vi "Generate Model.vi"(8 "error in (no error)":errorcluster, 11 "Velodyne 3D LIDAR in":refnum<class "Velodyne 3D LIDAR.lvclass">) -> (0 "error out":errorcluster, 3 "Velodyne 3D LIDAR out":refnum<class "Velodyne 3D LIDAR.lvclass">)   [LabVIEW 2017, in "NI_Robotics_Simulator.lvlib" / "Velodyne 3D LIDAR.lvclass"]
uses:
  <vilib>/robotics/Simulator/Plugin/Sensor/Velodyne 3D LIDAR/Velodyne 3D LIDAR.lvclass
  <vilib>/robotics/Simulator/Plugin/Sensor/Velodyne 3D LIDAR/Velodyne 3D LIDAR.lvclass/Velodyne 3D LIDAR.ctl
  <vilib>/robotics/Simulator/Robot Factory/Sensor/Base/ODESimulator_Base_Sensor.lvclass
  <vilib>/robotics/Simulator/3D-Physics/Sphere/3D_Physics_Sphere.lvclass
  c:/Program Files (x86)/National Instruments/LabVIEW 2017/vi.lib/robotics/Simulator/3D-Physics/Base/3D_Physics_Base.lvclass
  <vilib>/Utility/miscctls.llb/LV3DPointTypeDef.ctl
  <vilib>/robotics/Simulator/Robot Factory/Motor/ctl/Rate Joint.ctl
  <vilib>/robotics/Simulator/Robot Factory/Joint/Utilities/Joint Axis.ctl
  <vilib>/robotics/Simulator/Robot Factory/Motor/ODESimulator_Motor.lvclass
  <vilib>/Utility/xml.llb/Read From XML File(string).vi
  <vilib>/robotics/Simulator/3D-Physics/Base/3D_Physics_Base.lvclass
  <vilib>/robotics/Simulator/Robot Factory/Sensor/LIDAR/ODESimulator_LIDAR.lvclass
  <vilib>/robotics/Simulator/Robot Factory/Joint/ODESimulator_Joint.lvclass
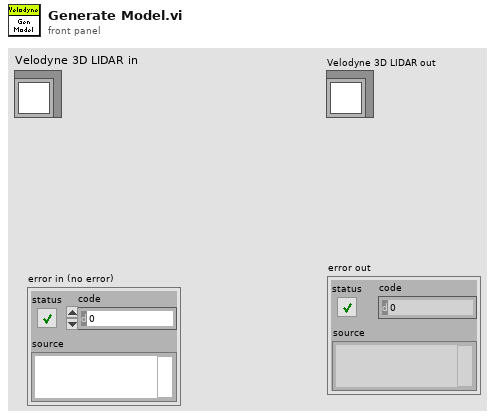
[diagram p1: front panel]
types:
  T1 = typedef "LV3DPointTypeDef.ctl" = cluster{"X":sgl, "Y":sgl, "Z":sgl}
  T2 = typedef "NI_Robotics_Simulator.lvlib/ODESimulator_Motor.lvclass/Rate Joint.ctl" = cluster{"ID":string, "Rate":dbl, "Axis":T3, "LVODE Joint":refnum<k20>}
  T3 = typedef "NI_Robotics_Simulator.lvlib/ODESimulator_Joint.lvclass/Joint Axis.ctl" = enum16{"Axis1", "Axis2", "Axis3"}
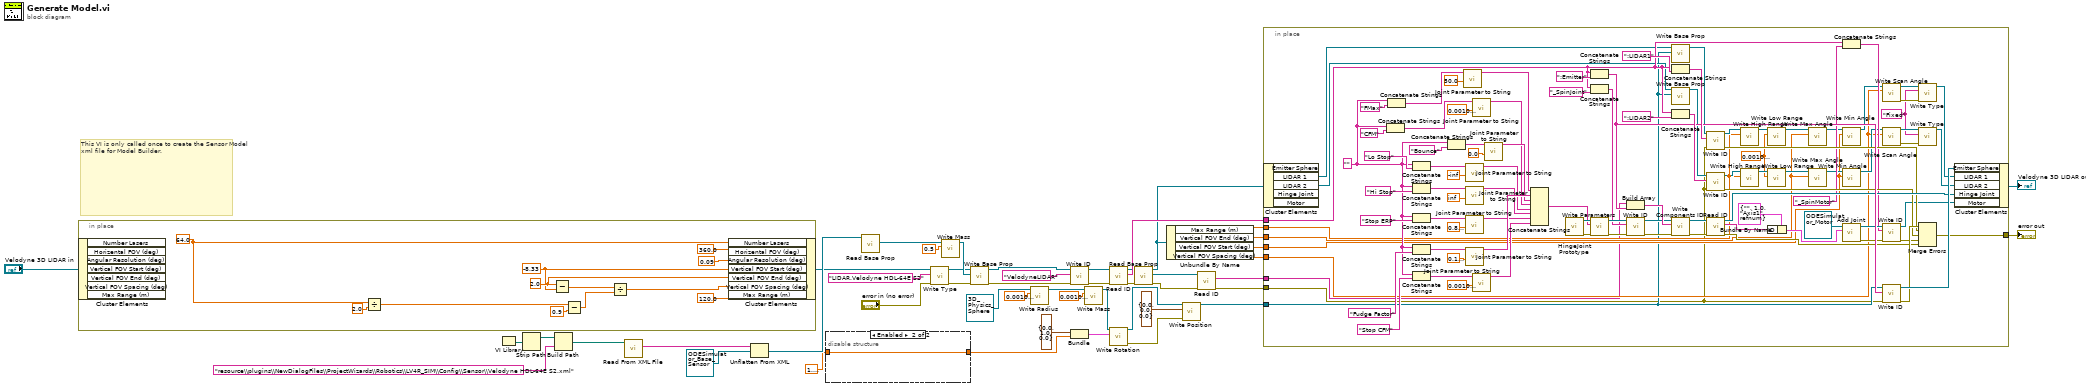
[diagram p0: block diagram]
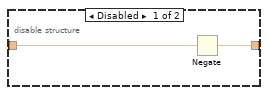
[diagram p2: hidden frame]
diagram:
  # "This VI is only called once to create the Sensor Model xml file for Model Builder."
  n1 = in-place {
    w57 = 2.0 ("Vertical FOV End (deg)")
    w56 = -8.33 ("Vertical FOV Start (deg)")
    w55 = 64.0 ("Number Lasers")
    n2 = in-place-cluster #1("Velodyne 3D LIDAR in") -> ()  [unwired: 7 out]
    n3 = Divide(x=w55, y=2.0) -> (x/y=w51:dbl)
    n4 = Subtract(x=w57, y=w56) -> (x-y=w53:dbl)
    n5 = Subtract(x=w51, y=0.9) -> (x-y=w50:dbl)
    n6 = Divide(x=w53, y=w50) -> (x/y=w52:dbl)
    n7 = in-place-cluster #1("Number Lasers"=w55, "Horizental FOV (deg)"=360.0, "Angular Resolution (deg)"=0.09, "Vertical FOV Start (deg)"=w56, "Vertical FOV End (deg)"=w57, "Vertical FOV Spacing (deg)"=w52, "Max Range (m)"=120.0) -> (w9:refnum<class "Velodyne 3D LIDAR.lvclass">)
  }
  n8 = VI Library() -> (path=w4:path)
  n9 = Strip Path(path=w4) -> (stripped path=w3:path)  [unwired: 1 out]
  n10 = Build Path(base path=w3, name or relative path="resource\\plugins\\NewDialogFiles\\ProjectWizards\\Robotics\\LV4R_SIM\\Config\\Sensor\\Velodyne HDL-64E S2.xml") -> (appended path=w1:path)
  n11 = call-poly <vilib>:"Read From XML File.vi"("XML File Path"=w1) -> ("XML Elements"=w39:string)  [unwired: 8 in, 2 out]
  n12 = Unflatten From XML(xml string=w39, type=refnum<class "ODESimulator_Base_Sensor.lvclass"> refnum ("NI_Robotics_Simulator.lvlib:ODESimulator_Base_Sensor.lvclass")) -> (value=w37:refnum<class "ODESimulator_Base_Sensor.lvclass">)  [unwired: 1 in, 1 out]
  n13 = disable-structure shown="Enabled" {
    disable-tunnel: 1.5707963267948966 -> [w62 w63]
    disable-tunnel: [w61 w63] -> w10
    frame Disabled {
      n14 = Negate(x=w62) -> (-x=w61:dbl)
    }
    frame Enabled {
    }
  }
  n15 = call-dynamic "Read Base Prop.vi"("ODESimulator_Base_Sensor in"=w37) -> ("NI_Robotics_Simulator.lvlib:3D_Physics_Base.lvclass"=w31:refnum<class "3D_Physics_Base.lvclass">)  [unwired: 8 in, 2 out]
  n16 = call-dynamic "Write Type.vi"("error in (no error)"="error in (no error)", "Type"="LIDAR.Velodyne HDL-64E S2", "ODESimulator_Base_Sensor in"=w9) -> ("error out"=w7:errorcluster, "ODESimulator_Base_Sensor out"=w8:refnum<class "Velodyne 3D LIDAR.lvclass">)  [unwired: 7 in]
  n17 = call-dynamic "Write Mass.vi"("Mass"=sgl 0.5, "Base in"=w31) -> ("Base out"=w29:refnum<class "3D_Physics_Base.lvclass">)  [unwired: 8 in, 1 out]
  n18 = call-dynamic "Write Base Prop.vi"("error in (no error)"=w7, "NI_Robotics_Simulator.lvlib:3D_Physics_Base.lvclass"=w29, "ODESimulator_Base_Sensor in"=w8) -> ("error out"=w34:errorcluster, "ODESimulator_Base_Sensor out"=w36:refnum<class "Velodyne 3D LIDAR.lvclass">)  [unwired: 7 in]
  n19 = call-dynamic "Write Radius.vi"("Radius"=sgl 0.001, "Sphere in"=refnum<class "3D_Physics_Sphere.lvclass"> refnum ("NI_Robotics_Simulator.lvlib:3D_Physics_Sphere")) -> ("Sphere out"=w24:refnum<class "3D_Physics_Sphere.lvclass">)  [unwired: 8 in, 1 out]
  n20 = call-dynamic "Write ID.vi"("error in (no error)"=w34, "ID"="VelodyneLIDAR", "Velodyne 3D LIDAR in"=w36) -> ("error out"=w32:errorcluster, "Velodyne 3D LIDAR out"=w35:refnum<class "Velodyne 3D LIDAR.lvclass">)  [unwired: 7 in]
  n21 = Bundle("Axis"=T1 {"X"=0.0, "Y"=1.0, "Z"=0.0}, w10) -> (w21:cluster{"Axis":T1, dbl})  [unwired: 1 in]
  n22 = call-dynamic "Write Mass.vi"("Mass"=sgl 0.001, "Base in"=w24) -> ("Base out"=w20:refnum<class "3D_Physics_Sphere.lvclass">)  [unwired: 8 in, 1 out]
  n23 = call-dynamic "Read ID.vi"("error in (no error)"=w32, "ODESimulator_Base_Sensor in"=w35) -> ("error out"=w46:errorcluster, "ID"=w48:string, "ODESimulator_Base_Sensor out"=w47:refnum<class "Velodyne 3D LIDAR.lvclass">)  [unwired: 7 in]
  n24 = call-dynamic "Write Rotation.vi"("Rotation"=w21, "Base in"=w20) -> ("error out"=w16:errorcluster, "Base out"=w19:refnum<class "3D_Physics_Sphere.lvclass">)  [unwired: 8 in]
  n25 = call-dynamic "Read Base Prop.vi"("error in (no error)"=w46, "ODESimulator_Base_Sensor in"=w47) -> ("error out"=w44:errorcluster, "NI_Robotics_Simulator.lvlib:3D_Physics_Base.lvclass"=w45:refnum<class "3D_Physics_Base.lvclass">, "ODESimulator_Base_Sensor out"=w28:refnum<class "Velodyne 3D LIDAR.lvclass">)  [unwired: 7 in]
  n26 = Unbundle By Name(w28) -> ("Max Range (m)"=w27:dbl, "Vertical FOV End (deg)"=w14:dbl, "Vertical FOV Start (deg)"=w13:dbl, "Vertical FOV Spacing (deg)"=w12:dbl)
  n27 = call-dynamic "Write Position.vi"("error in (no error)"=w16, "3D Point"=T1 {"X"=0.0, "Y"=0.0, "Z"=0.0}, "Base in"=w19) -> ("Base out"=w18:refnum<class "3D_Physics_Sphere.lvclass">)  [unwired: 7 in, 1 out]
  n28 = call-dynamic "Read ID.vi"("error in (no error)"=w44, "Base in"=w45) -> ("error out"=w41:errorcluster, "ID"=w43:string)  [unwired: 7 in, 1 out]
  n29 = in-place {
    in-place-border: w48 -> [w95]
    in-place-border: w43 -> [w64]
    in-place-border: w41 -> [w65]
    in-place-border: [w101] -> w40
    in-place-border: w27 -> [w78]
    in-place-border: w14 -> [w80]
    in-place-border: w13 -> [w81]
    in-place-border: w12 -> [w82]
    in-place-border: w18 -> [w66]
    w71 = "Fixed" ("Type")
    w79 = sgl 0.001 ("Low Range")
    w123 = "" ("string")
    n30 = in-place-cluster #2(w28) -> ("LIDAR 1"=w70:refnum<class "ODESimulator_LIDAR.lvclass">, "LIDAR 2"=w68:refnum<class "ODESimulator_LIDAR.lvclass">)  [unwired: 3 out]
    n31 = Concatenate Strings(w123, "CFM" ("Parameter Name")) -> (w149:string)
    n32 = Concatenate Strings(w123, "FMax" ("Parameter Name")) -> (w154:string)
    n33 = Concatenate Strings(w123, "Lo Stop" ("Parameter Name")) -> (w140:string)
    n34 = Concatenate Strings(w123, "Hi Stop" ("Parameter Name")) -> (w142:string)
    n35 = Concatenate Strings(w123, "Stop ERP" ("Parameter Name")) -> (w148:string)
    n36 = Concatenate Strings(w123, "Fudge Factor" ("Parameter Name")) -> (w152:string)
    n37 = Concatenate Strings(w123, "Stop CFM" ("Parameter Name")) -> (w146:string)
    n38 = Concatenate Strings(w123, "Bounce" ("Parameter Name")) -> (w151:string)
    n39 = call <vilib>:"Joint Parameter to String.vi"("dReal"=sgl 50.0, "Parameter Name"=w154) -> ("String"=w131:string)  [unwired: 9 in]
    n40 = call <vilib>:"Joint Parameter to String.vi"("dReal"=sgl -inf, "Parameter Name"=w140) -> ("String"=w124:string)  [unwired: 9 in]
    n41 = call <vilib>:"Joint Parameter to String.vi"("dReal"=sgl inf, "Parameter Name"=w142) -> ("String"=w127:string)  [unwired: 9 in]
    n42 = call <vilib>:"Joint Parameter to String.vi"("dReal"=sgl 0.8, "Parameter Name"=w148) -> ("String"=w126:string)  [unwired: 9 in]
    n43 = call <vilib>:"Joint Parameter to String.vi"("dReal"=sgl 0.1, "Parameter Name"=w152) -> ("String"=w130:string)  [unwired: 9 in]
    n44 = call <vilib>:"Joint Parameter to String.vi"("dReal"=sgl 0.001, "Parameter Name"=w149) -> ("String"=w128:string)  [unwired: 9 in]
    n45 = call <vilib>:"Joint Parameter to String.vi"("dReal"=sgl 0.001, "Parameter Name"=w146) -> ("String"=w125:string)  [unwired: 9 in]
    n46 = call <vilib>:"Joint Parameter to String.vi"("dReal"=sgl 0.0, "Parameter Name"=w151) -> ("String"=w129:string)  [unwired: 9 in]
    n47 = Concatenate Strings(w131, w130, w129, w128, w124, w127, w126, w125) -> (w120:string)
    n48 = call <vilib>:"HingeJoint Prototype.vi"() -> ("error out"=w121:errorcluster, "Joint out"=w122:refnum<class "ODESimulator_Joint.lvclass">)  [unwired: 10 in]
    n49 = Concatenate Strings(w95, ":Emitter") -> (w119:string)
    n50 = Concatenate Strings(w95, "_SpinJoint" ("string")) -> (w113:string)
    n51 = call-dynamic "Write Parameters.vi"("error in (no error)"=w121, "Parameters"=w120, "Joint in"=w122) -> ("error out"=w116:errorcluster, "Joint out"=w115:refnum<class "ODESimulator_Joint.lvclass">)  [unwired: 7 in]
    n52 = Build Array(w64, w119) -> (w118:string[])
    n53 = call-dynamic "Write ID.vi"("error in (no error)"=w116, "ID"=w113, "Joint in"=w115) -> ("error out"=w111:errorcluster, "Joint out"=w112:refnum<class "ODESimulator_Joint.lvclass">)  [unwired: 7 in]
    n54 = call-dynamic "Write Base Prop.vi"("NI_Robotics_Simulator.lvlib:3D_Physics_Base.lvclass"=w66, "ODESimulator_Base_Sensor in"=w70) -> ("ODESimulator_Base_Sensor out"=w69:refnum<class "ODESimulator_LIDAR.lvclass">)  [unwired: 8 in, 1 out]
    n55 = Concatenate Strings(w95, ":LIDAR1" ("string")) -> (w158:string)
    n56 = call-dynamic "Write Base Prop.vi"("NI_Robotics_Simulator.lvlib:3D_Physics_Base.lvclass"=w66, "ODESimulator_Base_Sensor in"=w68) -> ("ODESimulator_Base_Sensor out"=w67:refnum<class "ODESimulator_LIDAR.lvclass">)  [unwired: 8 in, 1 out]
    n57 = Concatenate Strings(w95, ":LIDAR2" ("string")) -> (w156:string)
    n58 = call-dynamic "Write Components ID.vi"("error in (no error)"=w111, "Components ID"=w118, "Joint in"=w112) -> ("error out"=w109:errorcluster, "Joint out"=w110:refnum<class "ODESimulator_Joint.lvclass">)  [unwired: 7 in]
    n59 = call-dynamic "Write ID.vi"("error in (no error)"=w65, "ID"=w158, "ODESimulator_Base_Sensor in"=w69) -> ("error out"=w104:errorcluster, "ODESimulator_Base_Sensor out"=w92:refnum<class "ODESimulator_LIDAR.lvclass">)  [unwired: 7 in]
    n60 = call-dynamic "Write ID.vi"("error in (no error)"=w65, "ID"=w156, "ODESimulator_Base_Sensor in"=w67) -> ("error out"=w103:errorcluster, "ODESimulator_Base_Sensor out"=w87:refnum<class "ODESimulator_LIDAR.lvclass">)  [unwired: 7 in]
    n61 = call-dynamic "Read ID.vi"("error in (no error)"=w109, "Joint in"=w110) -> ("error out"=w102:errorcluster, "ID"=w108:string, "Joint out"=w106:refnum<class "ODESimulator_Joint.lvclass">)  [unwired: 7 in]
    n62 = call-dynamic "Write High Range.vi"("High Range"=w78, "ODESimulator_LIDAR in"=w92) -> ("ODESimulator_LIDAR out"=w91:refnum<class "ODESimulator_LIDAR.lvclass">)  [unwired: 8 in, 1 out]
    n63 = call-dynamic "Write High Range.vi"("High Range"=w78, "ODESimulator_LIDAR in"=w87) -> ("ODESimulator_LIDAR out"=w86:refnum<class "ODESimulator_LIDAR.lvclass">)  [unwired: 8 in, 1 out]
    n64 = Bundle By Name(cluster=T2 {"ID"="", "Rate"=1.0, "Axis"=enum."Axis1", "LVODE Joint"=refnum} ("Rate Joint"), "ID"=w108) -> (w107:T2)
    n65 = call-dynamic "Write Low Range.vi"("Low Range"=w79, "ODESimulator_LIDAR in"=w91) -> ("ODESimulator_LIDAR out"=w90:refnum<class "ODESimulator_LIDAR.lvclass">)  [unwired: 8 in, 1 out]
    n66 = call-dynamic "Write Low Range.vi"("Low Range"=w79, "ODESimulator_LIDAR in"=w86) -> ("ODESimulator_LIDAR out"=w85:refnum<class "ODESimulator_LIDAR.lvclass">)  [unwired: 8 in, 1 out]
    n67 = call-dynamic "Write Max Angle.vi"("Max Angle"=w80, "ODESimulator_LIDAR in"=w90) -> ("ODESimulator_LIDAR out"=w89:refnum<class "ODESimulator_LIDAR.lvclass">)  [unwired: 8 in, 1 out]
    n68 = call-dynamic "Write Max Angle.vi"("Max Angle"=w80, "ODESimulator_LIDAR in"=w85) -> ("ODESimulator_LIDAR out"=w84:refnum<class "ODESimulator_LIDAR.lvclass">)  [unwired: 8 in, 1 out]
    n69 = Concatenate Strings(w95, "_SpinMotor" ("string")) -> (w93:string)
    n70 = call-dynamic "Write Min Angle.vi"("Min Angle"=w81, "ODESimulator_LIDAR in"=w89) -> ("ODESimulator_LIDAR out"=w88:refnum<class "ODESimulator_LIDAR.lvclass">)  [unwired: 8 in, 1 out]
    n71 = call-dynamic "Write Min Angle.vi"("Min Angle"=w81, "ODESimulator_LIDAR in"=w84) -> ("ODESimulator_LIDAR out"=w83:refnum<class "ODESimulator_LIDAR.lvclass">)  [unwired: 8 in, 1 out]
    n72 = call-dynamic "Add Joint.vi"("Rate Joint"=w107, "Motor in"=refnum<class "ODESimulator_Motor.lvclass"> refnum) -> ("error out"=w97:errorcluster, "Motor out"=w99:refnum<class "ODESimulator_Motor.lvclass">)  [unwired: 8 in]
    n73 = call-dynamic "Write Scan Angle.vi"("Scan Angle"=w82, "ODESimulator_LIDAR in"=w88) -> ("error out"=w76:errorcluster, "ODESimulator_LIDAR out"=w77:refnum<class "ODESimulator_LIDAR.lvclass">)  [unwired: 8 in]
    n74 = call-dynamic "Write Scan Angle.vi"("Scan Angle"=w82, "ODESimulator_LIDAR in"=w83) -> ("error out"=w74:errorcluster, "ODESimulator_LIDAR out"=w73:refnum<class "ODESimulator_LIDAR.lvclass">)  [unwired: 8 in]
    n75 = call-dynamic "Write ID.vi"("error in (no error)"=w97, "ID"=w93, "Motor in"=w99) -> ("error out"=w96:errorcluster, "Motor out"=w98:refnum<class "ODESimulator_Motor.lvclass">)  [unwired: 7 in]
    n76 = call-dynamic "Write ID.vi"("error in (no error)"=w65, "ID"=w119, "Base in"=w66) -> ("error out"=w105:errorcluster, "Base out"=w160:refnum<class "3D_Physics_Sphere.lvclass">)  [unwired: 7 in]
    n77 = call-dynamic "Write Type.vi"("error in (no error)"=w76, "Type"=w71, "ODESimulator_Base_Sensor in"=w77) -> ("ODESimulator_Base_Sensor out"=w75:refnum<class "ODESimulator_LIDAR.lvclass">)  [unwired: 7 in, 1 out]
    n78 = call-dynamic "Write Type.vi"("error in (no error)"=w74, "Type"=w71, "ODESimulator_Base_Sensor in"=w73) -> ("ODESimulator_Base_Sensor out"=w72:refnum<class "ODESimulator_LIDAR.lvclass">)  [unwired: 7 in, 1 out]
    n79 = Merge Errors(w105, w104, w103, w96, w102) -> (w101:errorcluster)
    n80 = in-place-cluster #2("Emitter Sphere"=w160, "LIDAR 1"=w75, "LIDAR 2"=w72, "Hinge Joint"=w106, "Motor"=w98) -> (→"Velodyne 3D LIDAR out":refnum<class "Velodyne 3D LIDAR.lvclass">)
  }
  "error out" <- w40
